vi "Set Baud Rate.vi"(8 "error in":errorcluster, 10 "Baud Rate":T1(ring), 11 "ICAN in":refnum<class "ICAN.lvclass">) -> (0 "error out":errorcluster, 3 "ICAN out":refnum<class "ICAN.lvclass">)   [LabVIEW 2023, in "ICAN.lvclass"]
uses:
  ICAN.lvclass
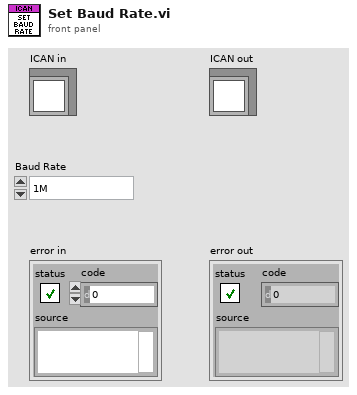
[diagram p1: front panel]
types:
  T1 = enum16{"1M", "800k", "500k", "250k", "125k", "50k", "25k", "10k"}
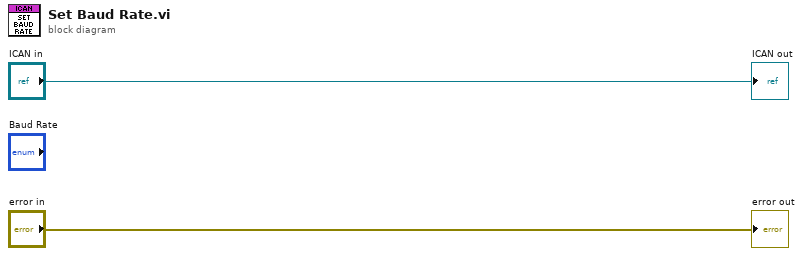
[diagram p0: block diagram]
diagram:
  "error out" <- "error in"
  "ICAN out" <- "ICAN in"
